vi "Test Adquisition API.vi"() -> ()   [LabVIEW 2020]
doc: "Adquisition API Tester."
uses:
  Adquisition.lvlib
panel:
  in  "wait for reply":bool=TRUE
  in  "Show Block Diagram":bool
  in  "X":dbl=1.0
  out "Reply Payload":dbl
  in  "Stop Module":bool
  in  "Start Module":bool
  out "Do Something Count":i32
  in  "Test Do Something Else and Wait for Reply":bool
  in  "Hide Module Panel":bool
  in  "Show Module Panel":bool
  in  "Test Do Something Else":bool
  in  "Test Do Something":bool
  out "Status":string
  out "Module Running?":bool
  # "This VI tests the API for the Module."
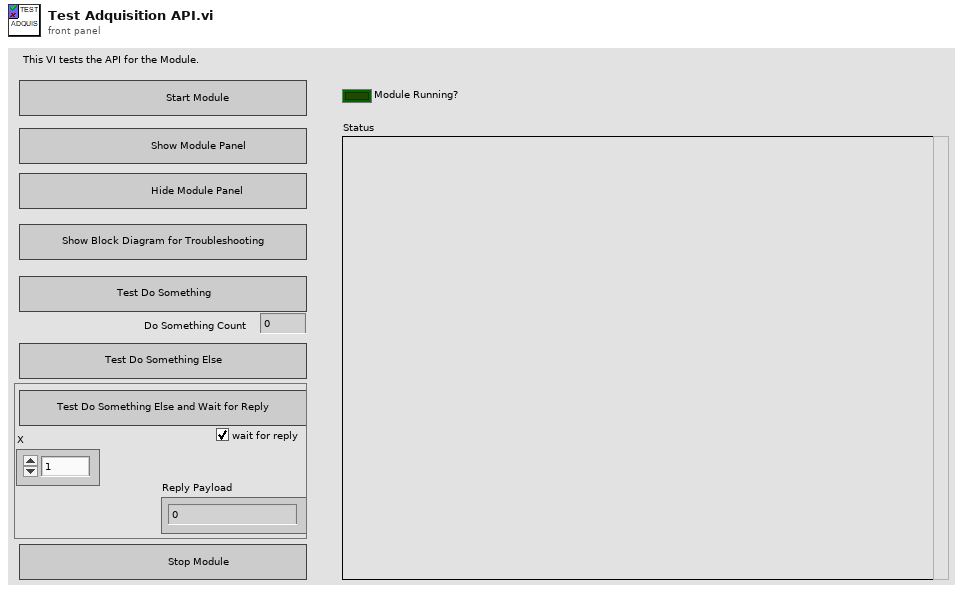
[diagram p1: front panel]
types:
  T1 = typedef "Adquisition.lvlib/Broadcast Events--cluster.ctl" = cluster{"Module Did Init":refnum<user-event>, "Status Updated":refnum<user-event>, "Error Reported":refnum<user-event>, "Did Something":refnum<user-event>, "Module Did Stop":refnum<user-event>, "Update Module Execution Status":refnum<user-event>}
  T2 = typedef "Adquisition.lvlib/Do Something Else and Wait (Reply Payload)--cluster.ctl" = cluster{"Value":dbl, "error":errorcluster}
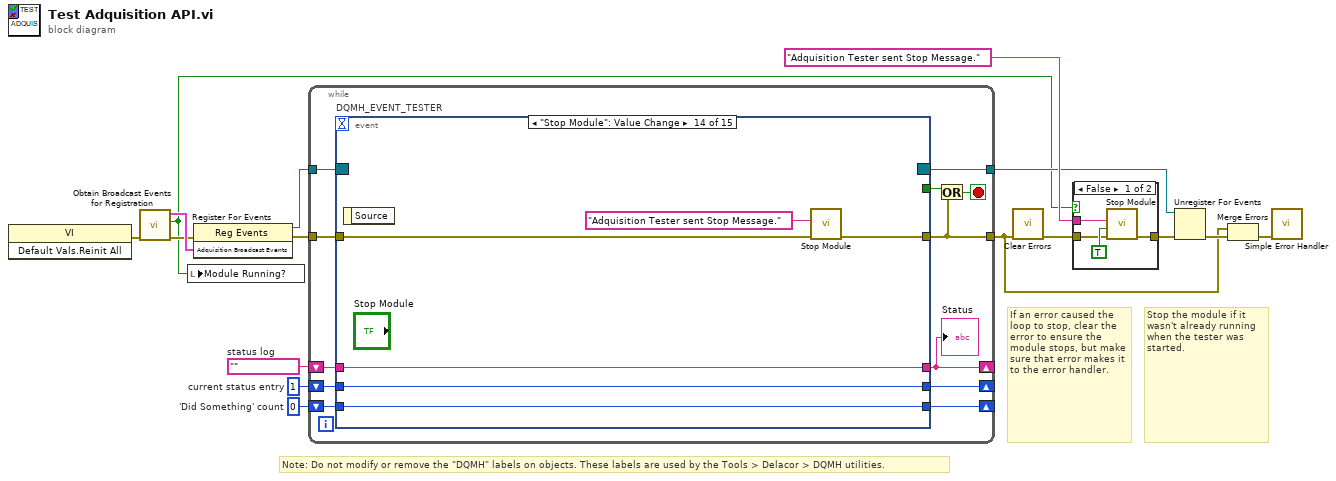
[diagram p0: block diagram]
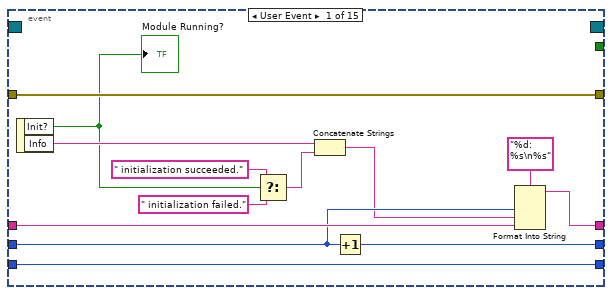
[diagram p3: hidden frame]
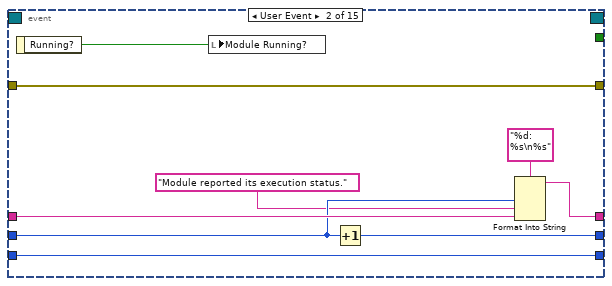
[diagram p4: hidden frame]
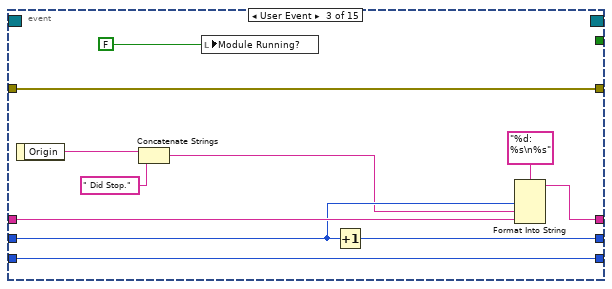
[diagram p5: hidden frame]
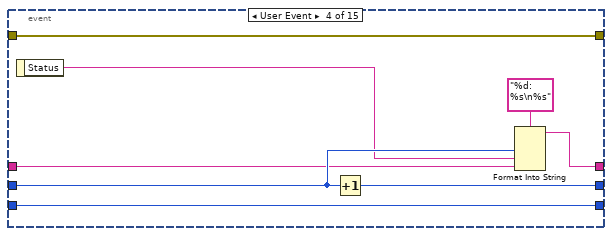
[diagram p6: hidden frame]
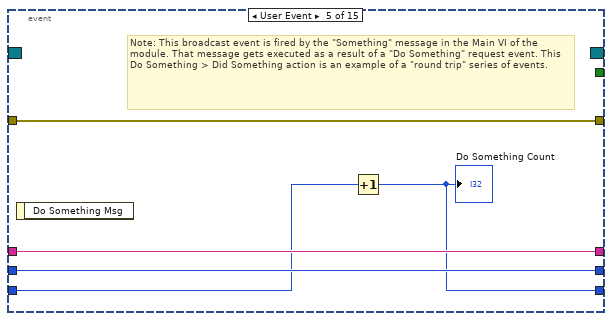
[diagram p7: hidden frame]
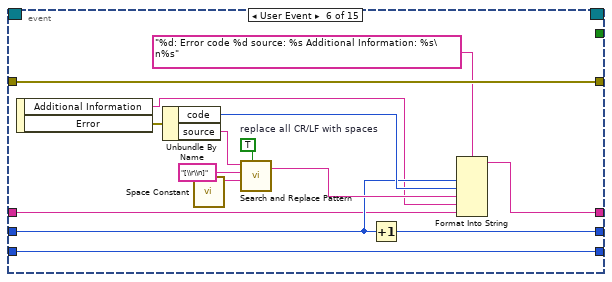
[diagram p8: hidden frame]
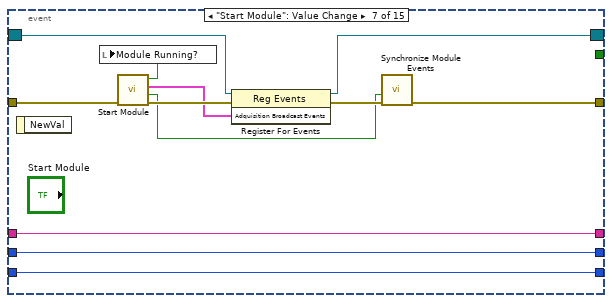
[diagram p9: hidden frame]
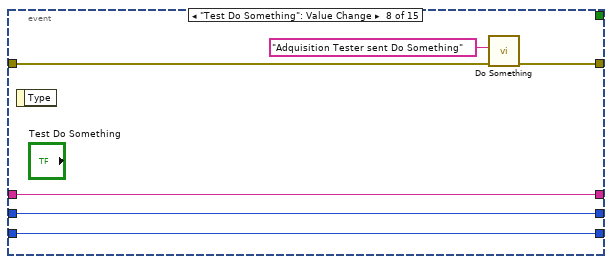
[diagram p10: hidden frame]
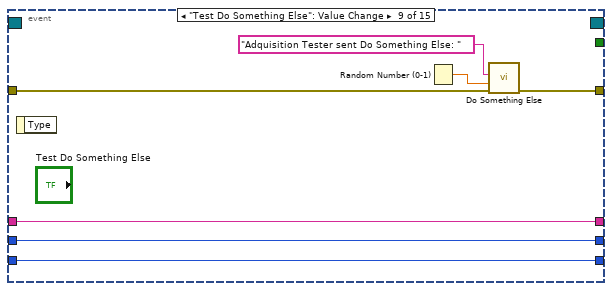
[diagram p11: hidden frame]
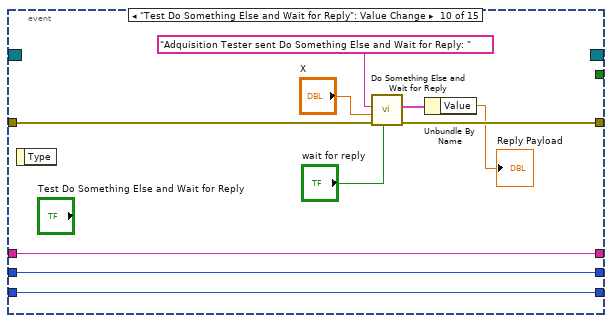
[diagram p12: hidden frame]
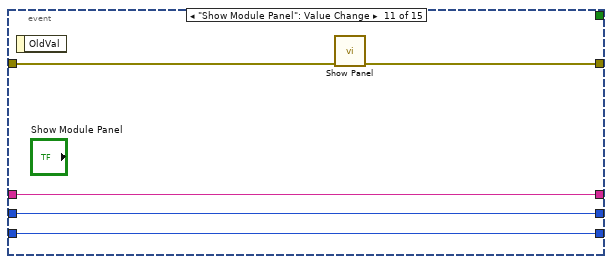
[diagram p13: hidden frame]
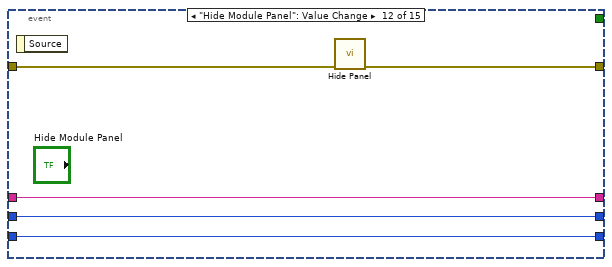
[diagram p14: hidden frame]
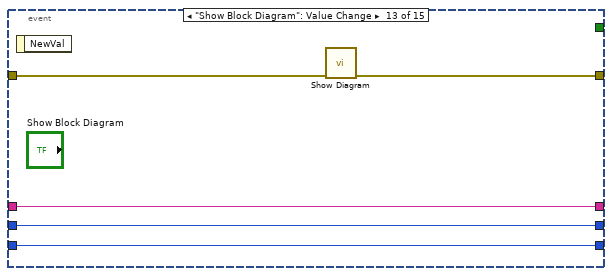
[diagram p15: hidden frame]
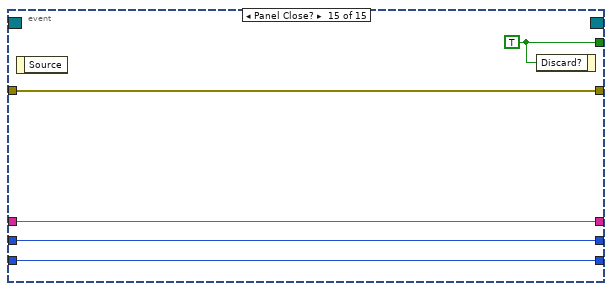
[diagram p16: hidden frame]
diagram:
  w11 = 0  # 'Did Something' count
  w12 = 1  # current status entry
  w13 = ""  # status log
  # "Stop the module if it wasn't already running when the tester was started."
  # "If an error caused the loop to stop, clear the error to ensure the module stops, but make sure that error makes it to the error handler."
  # "Note: Do not modify or remove the \"DQMH\" labels on objects. These labels are used by the Tools > Delacor > DQMH utilities."
  n1 = invoke class="VI" method="Default Vals.Reinit All"() -> (error out=w3:errorcluster)  [unwired: 3 in, 2 out]
  n2 = call "Obtain Broadcast Events for Registration.vi"("error in (no error)"=w3) -> ("error out"=w2:errorcluster, "Already running?"=w1:bool, "Adquisition Broadcast Events"=w9:T1)  [unwired: 8 in]
  n3 = local write "Module Running?"(w1) -> ()
  n4 = register-events(error in=w2, w9) -> (reference out=w8:refnum<event-registration>, error out=w10:errorcluster)  [unwired: 1 in]
  n5 = while {
    tunnel: w8 -> [w28]
    tunnel: [w17] -> w4
    shift-right: [w23] -> _
    shift-left: w13 -> [w25]
    shift-right: [w24] -> _
    shift-left: w12 -> [w26]
    shift-right: [w21] -> _
    shift-left: w11 -> [w22]
    tunnel: w10 -> [w19]
    tunnel: [w18] -> w7
    stop <- w20 stop-if-true
    n6 = event "DQMH_EVENT_TESTER" shown="[13] \"Stop Module\": Value Change" {
      selector: w28 -> [_ _ _ _ _ _ w94 _ _ _ _ _ _ _ _]
      dyn-events: [_ _ _ _ _ _ w93 _ _ _ _ _ _ _ _] -> w18
      timeout: _ -> [_ _ _ _ _ _ _ _ _ _ _ _ _ _ _]
      tunnel: [_ _ _ _ _ _ _ _ _ _ _ _ _ _ w150] -> w27
      tunnel: [w41 w43 w51 w62 w70 w88 w92 w107 w114 w124 w129 w134 w135 w142 w146] -> w17
      tunnel: w26 -> [w38 w48 w59 w66 w73 w78 w98 w104 w110 w121 w127 w132 w137 w144 w148]
      tunnel: w25 -> [w39 w49 w60 w65 w74 w76 w99 w105 w111 w122 w128 w133 w138 w145 w149]
      tunnel: [w36 w46 w57 w67 w74 w79 w99 w105 w111 w122 w128 w133 w138 w145 w149] -> w23
      tunnel: [w37 w47 w58 w69 w73 w77 w98 w104 w110 w121 w127 w132 w137 w144 w148] -> w24
      tunnel: w22 -> [w33 w44 w53 w63 w72 w89 w97 w103 w109 w120 w126 w131 w136 w143 w147]
      tunnel: [w33 w44 w53 w63 w71 w89 w97 w103 w109 w120 w126 w131 w136 w143 w147] -> w21
      tunnel: w19 -> [w41 w43 w51 w62 w70 w88 w91 w102 w108 w117 w125 w130 w139 w140 w146]
      event User Event {
        n7 = event-data() -> ("Init?"=w32:bool, "Info"=w35:string)  [unwired: 1 in]
        "Module Running?" <- w32
        n8 = Select(t=" initialization succeeded.", s=w32, f=" initialization failed.") -> (s? t:f=w29:string)
        n9 = Concatenate Strings(w35, w29) -> (w34:string)
        n10 = Increment(x=w38) -> (x+1=w37:i32)
        n11 = Format Into String(format string="%d: %s\n%s", w38, w34, w39) -> (resulting string=w36:string)  [unwired: 2 in, 1 out]
      }
      event User Event {
        n12 = event-data() -> ("Running?"=w42:bool)  [unwired: 1 in]
        n13 = local write "Module Running?"(w42) -> ()
        n14 = Increment(x=w48) -> (x+1=w47:i32)
        n15 = Format Into String(format string="%d: %s\n%s", w48, "Module reported its execution status.", w49) -> (resulting string=w46:string)  [unwired: 2 in, 1 out]
      }
      event User Event {
        n16 = event-data() -> ("Origin"=w56:string)  [unwired: 1 in]
        n17 = Concatenate Strings(w56, " Did Stop.") -> (w55:string)
        n18 = local write "Module Running?"(FALSE ("Module Did Init?")) -> ()
        n19 = Increment(x=w59) -> (x+1=w58:i32)
        n20 = Format Into String(format string="%d: %s\n%s", w59, w55, w60) -> (resulting string=w57:string)  [unwired: 2 in, 1 out]
      }
      event User Event {
        n21 = event-data() -> ("Status"=w64:string)  [unwired: 1 in]
        n22 = Increment(x=w66) -> (x+1=w69:i32)
        n23 = Format Into String(format string="%d: %s\n%s", w66, w64, w65) -> (resulting string=w67:string)  [unwired: 2 in, 1 out]
      }
      event User Event {
        # "Note: This broadcast event is fired by the \"Something\" message in the Main VI of the module. That message gets executed as a result of a \"Do Something\" request event. This Do Something > Did Something action is an example of a \"round trip\" series of events."
        n24 = event-data() -> ()  [unwired: 1 in, 1 out]
        n25 = Increment(x=w72) -> (x+1=w71:i32)
        "Do Something Count" <- w71
      }
      event User Event {
        w84 = TRUE  # replace all CR/LF with spaces
        n26 = event-data() -> ("Additional Information"=w75:string, "Error"=w80:errorcluster)  [unwired: 1 in]
        n27 = Unbundle By Name(w80) -> ("code"=w81:i32, "source"=w82:string)
        n28 = call <vilib>:"Space Constant.vi"() -> ("String"=w85:string)
        n29 = call <vilib>:"Search and Replace Pattern.vi"("string"=w82, "regular expression (\"\")"="[\\r\\n]" ("regular expression (\"\")"), "replace string (\"\")"=w85, "replace all? (F)"=w84) -> ("result string"=w83:string)  [unwired: 1 in, 1 out]
        n30 = Increment(x=w78) -> (x+1=w77:i32)
        n31 = Format Into String(format string="%d: Error code %d source: %s Additional Information: %s\n%s", w78, w81, w83, w75, w76) -> (resulting string=w79:string)  [unwired: 2 in, 1 out]
      }
      event "Start Module": Value Change {
        n32 = event-data() -> ()  [unwired: 1 in, 1 out]
        n33 = call "Start Module.vi"("error in (no error)"=w91) -> ("error out"=w100:errorcluster, "Wait for Event Sync?"=w96:bool, "Adquisition Broadcast Events"=w95:T1, "Module Was Already Running?"=w90:bool)  [unwired: 7 in]
        n34 = local write "Module Running?"(w90) -> ()
        n35 = register-events(reference=w94, error in=w100, w95) -> (reference out=w93:refnum<event-registration>, error out=w101:errorcluster)
        n36 = call "Synchronize Module Events.vi"("error in (no error)"=w101, "Wait for Event Sync?"=w96) -> ("error out"=w92:errorcluster)  [unwired: 9 in]
      }
      event "Test Do Something": Value Change {
        n37 = event-data() -> ()  [unwired: 1 in, 1 out]
        n38 = call "Do Something.vi"("error in (no error)"=w102, "Do Something Message"="Adquisition Tester sent Do Something") -> ("error out"=w107:errorcluster)  [unwired: 9 in]
      }
      event "Test Do Something Else": Value Change {
        n39 = event-data() -> ()  [unwired: 1 in, 1 out]
        n40 = Random Number (0-1)() -> (number: 0 to 1=w112:dbl)
        n41 = call "Do Something Else.vi"("error in (no error)"=w108, "X"=w112, "Do Something Else Message"="Adquisition Tester sent Do Something Else: " ("Do Something Message")) -> ("error out"=w114:errorcluster)  [unwired: 8 in]
      }
      event "Test Do Something Else and Wait for Reply": Value Change {
        n42 = event-data() -> ()  [unwired: 1 in, 1 out]
        n43 = call "Do Something Else and Wait for Reply.vi"("wait for reply (T)"="wait for reply", "error in (no error)"=w117, "X"="X", "Do Something Else Message"="Adquisition Tester sent Do Something Else and Wait for Reply: " ("Do Something Message")) -> ("error out"=w124:errorcluster, "Reply Payload"=w119:T2)  [unwired: 5 in, 1 out]
        n44 = Unbundle By Name(w119) -> ("Value"=→"Reply Payload":dbl)
      }
      event "Show Module Panel": Value Change {
        n45 = event-data() -> ()  [unwired: 1 in, 1 out]
        n46 = call "Show Panel.vi"("error in (no error)"=w125) -> ("error out"=w129:errorcluster)  [unwired: 10 in]
      }
      event "Hide Module Panel": Value Change {
        n47 = event-data() -> ()  [unwired: 1 in, 1 out]
        n48 = call "Hide Panel.vi"("error in (no error)"=w130) -> ("error out"=w134:errorcluster)  [unwired: 10 in]
      }
      event "Show Block Diagram": Value Change {
        n49 = event-data() -> ()  [unwired: 1 in, 1 out]
        n50 = call "Show Diagram.vi"("error in (no error)"=w139) -> ("error out"=w135:errorcluster)  [unwired: 10 in]
      }
      event "Stop Module": Value Change {
        n51 = event-data() -> ()  [unwired: 1 in, 1 out]
        n52 = call "Stop Module.vi"("error in (no error)"=w140, "Origin"="Adquisition Tester sent Stop Message.") -> ("error out"=w142:errorcluster)  [unwired: 9 in]
      }
      event Panel Close? {
        w150 = TRUE ("Discard?")
        n53 = event-data() -> ()  [unwired: 1 in, 1 out]
        n54 = event-data("Discard?"=w150) -> ()  [unwired: 1 in, 1 out]
      }
    }
    "Status" <- w23
    n55 = Or(x=w27, y=w17) -> (x .or. y?=w20:bool)
  }
  n56 = call <vilib>:"Clear Errors.vi"("error in (no error)"=w4) -> ("error out"=w6:errorcluster)  [unwired: 5 in, 1 out]
  n57 = case shown="False" w1 {
    tunnel: [w154 w155] -> w15
    tunnel: "Adquisition Tester sent Stop Message." ("Origin") -> [w153 _]
    tunnel: w6 -> [w151 w155]
    frame False {
      n58 = call "Stop Module.vi"("error in (no error)"=w151, "Wait for Module to Stop? (F)"=TRUE ("Wait for Module to stop?"), "Origin"=w153) -> ("error out"=w154:errorcluster)  [unwired: 8 in]
    }
    frame True {
    }
  }
  n59 = Unregister For Events(event registration refnum=w7, error in=w15) -> (error out=w16:errorcluster)
  n60 = Merge Errors(w4, w16) -> (w5:errorcluster)
  n61 = call <vilib>:"Simple Error Handler.vi"("error in (no error)"=w5) -> ()  [unwired: 4 in, 5 out]
